vi "SimulatedConfigRefGlobal.vi"() -> ()   [LabVIEW 2017, in "CmsAcquisition.lvlib"]
uses:
  <vilib>/addons/InsightCM/Devices/Shared/Cms/CmsAcquisition/CmsAcquisition.lvlib
  <vilib>/addons/InsightCM/Devices/Shared/Cms/CmsAcquisition/controls/AcqSimulated_ConfigRefs.ctl
panel:
  out "HideUI":bool
  in  "Rule 2":refnum<vi>
  in  "Rule":refnum<vi>
  in  "Short":refnum<vi>
  in  "Open":refnum<vi>
  in  "SimConfigRefs":T1
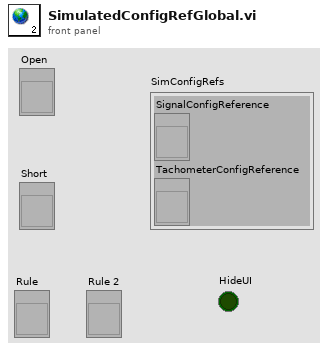
[diagram p1: front panel]
types:
  T1 = typedef "CmsAcquisition.lvlib/AcqSimulated_ConfigRefs.ctl" = cluster{"SignalConfigReference":refnum<vi>, "TachometerConfigReference":refnum<vi>}
diagram:
